vi "Stop Core.vi"(10 "final error code":i32, 11 "Client in":refnum<class "Client.lvclass">=refnum) -> (3 "Client out":refnum<class "Client.lvclass">)   [LabVIEW 2023, in "Client.lvlib" / "Client.lvclass"]
doc: "(<B>Filename</B>: Actor Framework.lvlib:Actor.lvclass:Stop Core.vi)\n\nDefines what the actor does before it stops. Use the <B>final error code</B> input to determine whether the actor shut down in response to an error.\n\nBy default, this method passes the Stop message along to all auto-stop nested actors. A descendant class may override this method to define additional behavior, such as shutting down any processes the actor initiated in its override of the Actor Core method."
uses:
  Client.lvclass
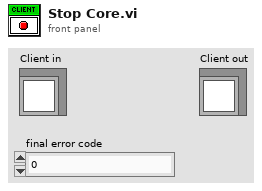
[diagram p1: front panel]
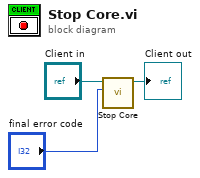
[diagram p0: block diagram]
diagram:
  n1 = call-parent "Stop Core.vi"("final error code"="final error code", "Actor in"="Client in") -> ("Actor out"=→"Client out":refnum<class "Client.lvclass">)  [unwired: 9 in]
